vi "GV_LegendOnOff.vi"(8 "error in (no error)":errorcluster, 9 "On?":bool, 11 "Gviewer in":refnum<class "Gviewer.lvclass">) -> (0 "error out":errorcluster, 1 "Visible?":bool, 3 "Gviewer out":refnum<class "Gviewer.lvclass">)   [LabVIEW 2020, in "Sgraph_lib_V1.lvlib" / "Gviewer.lvclass"]
doc: "Andre Koelewijn, 27 April 2021,\n\nSet Legend to be shown or hidden"
uses:
  Gviewer.lvclass
  Gviewer.lvclass/Gviewer.ctl
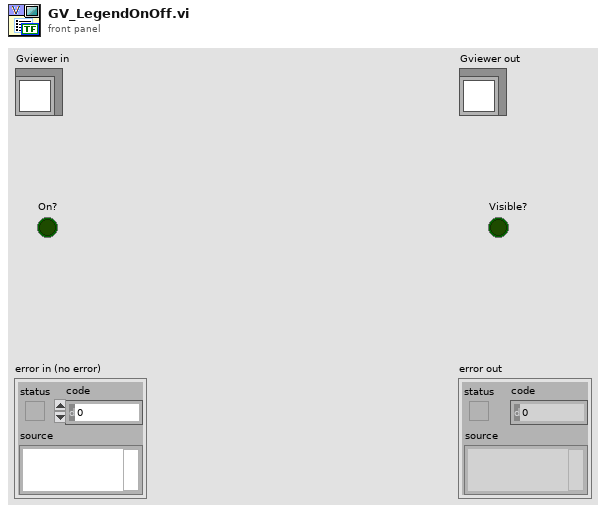
[diagram p1: front panel]
types:
  T1 = typedef "LVPositionTypeDef.ctl" = cluster{"Left":i32, "Top":i32}
  T2 = typedef "LVBoundsTypeDef.ctl" = cluster{"Width":u32, "Height":u32}
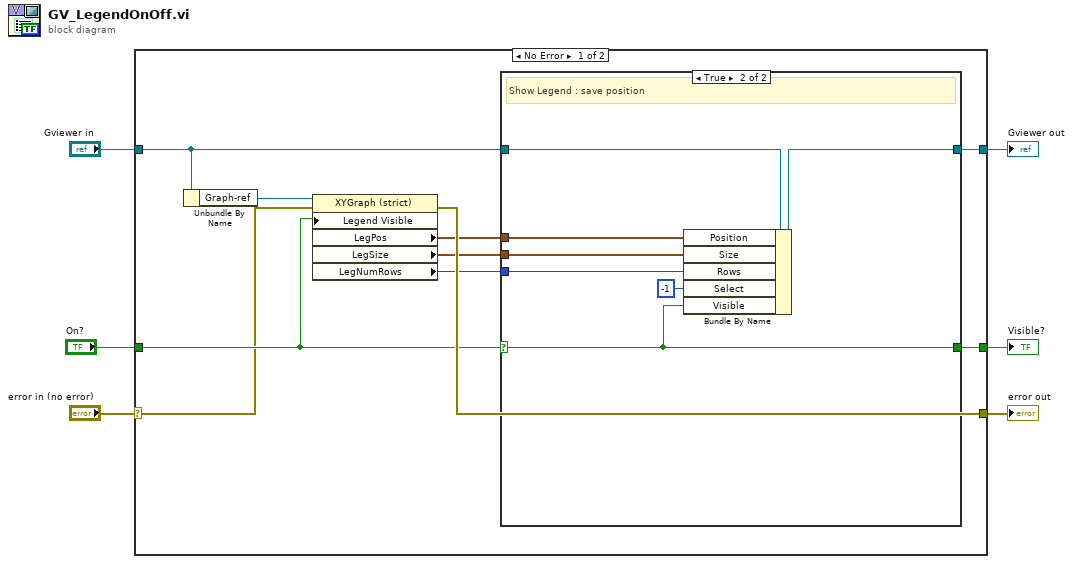
[diagram p0: block diagram]
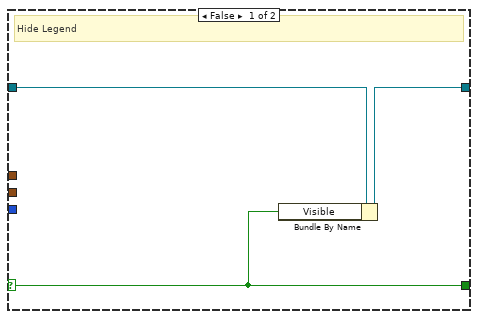
[diagram p2: hidden frame]
diagram:
  n1 = case shown="No Error" "error in (no error)" {
    selector: "error in (no error)" -> [w7 w28]
    tunnel: [w16 w28] -> w5
    tunnel: [w13 w27] -> w3
    tunnel: "Gviewer in" -> [w14 w27]
    tunnel: [w15 _] -> w2
    tunnel: "On?" -> [w9 _]
    frame No Error {
      n2 = Unbundle By Name(w14) -> ("Graph-ref"=w8:refnum<vi>)
      n3 = property class="XYGraph (strict)"(reference=w8, error in=w7, "Legend Visible"=w9) -> (error out=w16:errorcluster, "LegPos"=w12:T1, "LegSize"=w11:T2, "LegNumRows"=w10:u32)  [unwired: 1 out]
      n4 = case shown="True" w9 {
        selector: w9 -> [w19 w20]
        tunnel: [w19 w20] -> w15
        tunnel: w14 -> [w17 w25]
        tunnel: [w18 w26] -> w13
        tunnel: w12 -> [_ w24]
        tunnel: w11 -> [_ w23]
        tunnel: w10 -> [_ w22]
        frame False {
          # "Hide Legend"
          n5 = Bundle By Name(cluster=w17, "Visible"=w19) -> (w18:refnum<class "Gviewer.lvclass">)
        }
        frame True {
          # "Show Legend : save position"
          n6 = Bundle By Name(cluster=w25, "Position"=w24, "Size"=w23, "Rows"=w22, "Select"=-1 ("Legend.Select"), "Visible"=w20) -> (w26:refnum<class "Gviewer.lvclass">)
        }
      }
    }
    frame Error {
    }
  }
  "error out" <- w5
  "Gviewer out" <- w3
  "Visible?" <- w2
